vi "S7Com_ISO_READ(SubVI).vi"(4 "error in":errorcluster, 5 "timeout ms (25000)":i32, 7 "connection ID in":refnum<k5>) -> (0 "error out":errorcluster, 1 "Error":bool, 2 "TPDU Data":T1 format="X%02x", 3 "connection ID out":refnum<k5>)   [LabVIEW 2019]
doc: "Reads the Transport Data Unit (TDU) and strips the ISO 8073 Header."
uses:
  S7Com_HexByteArray.ctl
  S7Com_HexByte.ctl
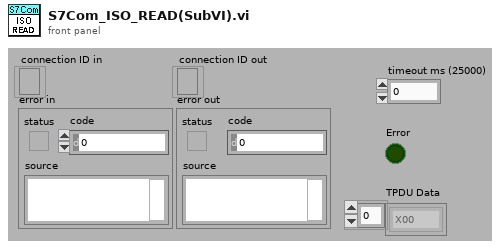
[diagram p1: front panel]
types:
  T1 = typedef "S7Com_HexByteArray.ctl" = T2[]
  T2 = typedef "S7Com_HexByte.ctl" = u8
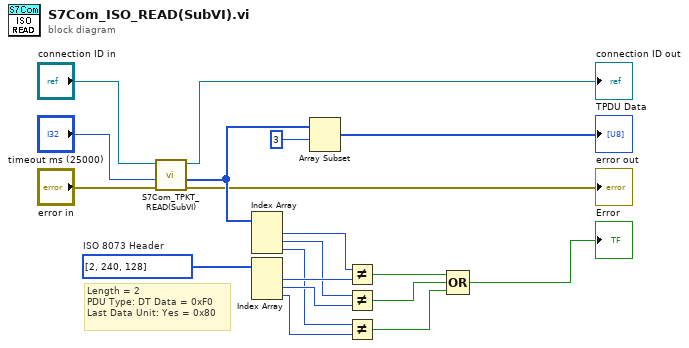
[diagram p0: block diagram]
diagram:
  w2 = u8[] [2, 240, 128]  # ISO 8073 Header
  # "Length = 2\nPDU Type: DT Data = 0xF0\nLast Data Unit: Yes = 0x80"
  n1 = call "S7Com_TPKT_READ(SubVI).vi"("error in"="error in", "timeout ms (25000)"="timeout ms (25000)", "connection ID in"="connection ID in") -> ("error out"=→"error out":errorcluster, "TPDU Data"=w6:T1, "connection ID out"=→"connection ID out":refnum<k5>)  [unwired: 2 out]
  n2 = Index Array(array=w6) -> (element #1=w16:T2, element #2=w14:T2, element #3=w12:T2)  [unwired: 3 in]
  n3 = Index Array(array=w2) -> (element #1=w15:u8, element #2=w13:u8, element #3=w11:u8)  [unwired: 3 in]
  n4 = Array Subset(array=w6, index=3 ("length")) -> (→"TPDU Data":T1)  [unwired: 1 in]
  n5 = Not Equal?(x=w16, y=w15) -> (x != y?=w9:bool)
  n6 = Not Equal?(x=w14, y=w13) -> (x != y?=w10:bool)
  n7 = Not Equal?(x=w12, y=w11) -> (x != y?=w8:bool)
  n8 = Compound Arithmetic op=OR(w9, w10, w8) -> (→"Error":bool)
